vi "getStateName.vi"(9 "error in (no error)":errorcluster, 11 "configurable in":refnum<class "configurable.lvclass">) -> (1 "error out":errorcluster, 2 "State Name":string, 3 "configurable out":refnum<class "configurable.lvclass">)   [LabVIEW 2020, in "eos.lvlib" / "configurable.lvclass"]
uses:
  configurable.lvclass
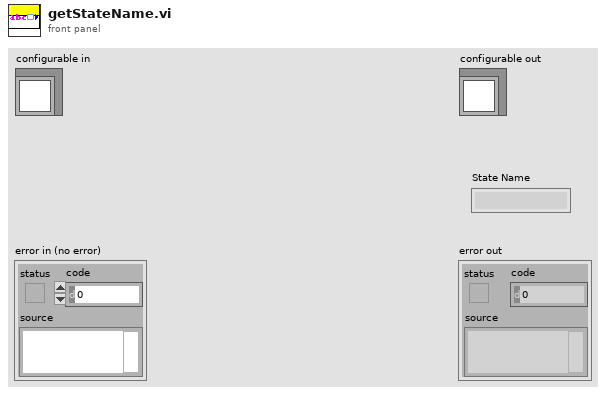
[diagram p1: front panel]
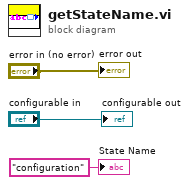
[diagram p0: block diagram]
diagram:
  "error out" <- "error in (no error)"
  "configurable out" <- "configurable in"
  "State Name" <- "configuration" ("State Name")
